vi "READ MODBUS DATA.vi"() -> ()   [LabVIEW 2025]
uses:
  <vilib>/NI/Modbus Library/API/Wrapper/Create TCP Master.vi
  <vilib>/NI/Modbus Library/API/Master/Modbus Master.lvclass
  <vilib>/NI/Modbus Library/API/Wrapper/API Main.lvlib
panel:
  out "Data Register":u16[](array[numeric])
  out "8":sgl
  out "7":sgl
  out "6":sgl
  out "5":sgl
  out "4":sgl
  out "3":sgl
  out "2":sgl
  out "1":sgl
  out "error out":errorcluster
  in  "Stop":bool
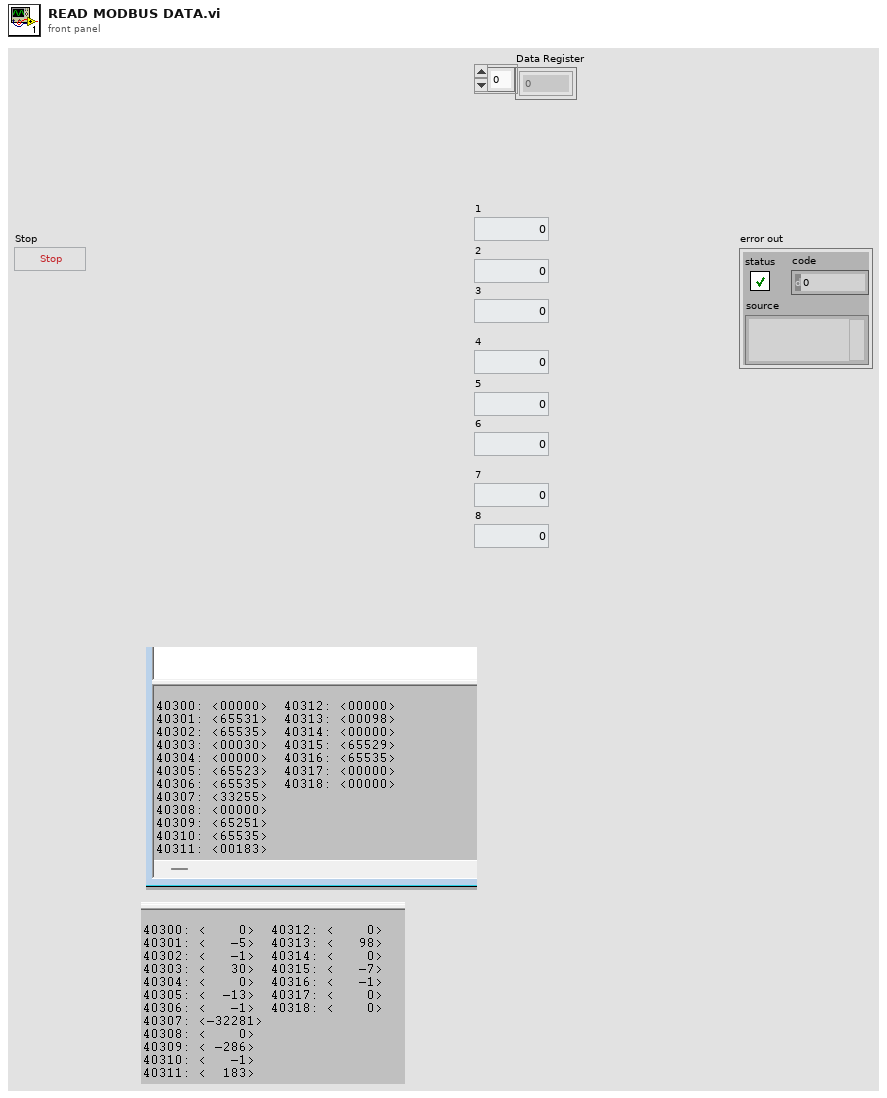
[diagram p1: front panel]
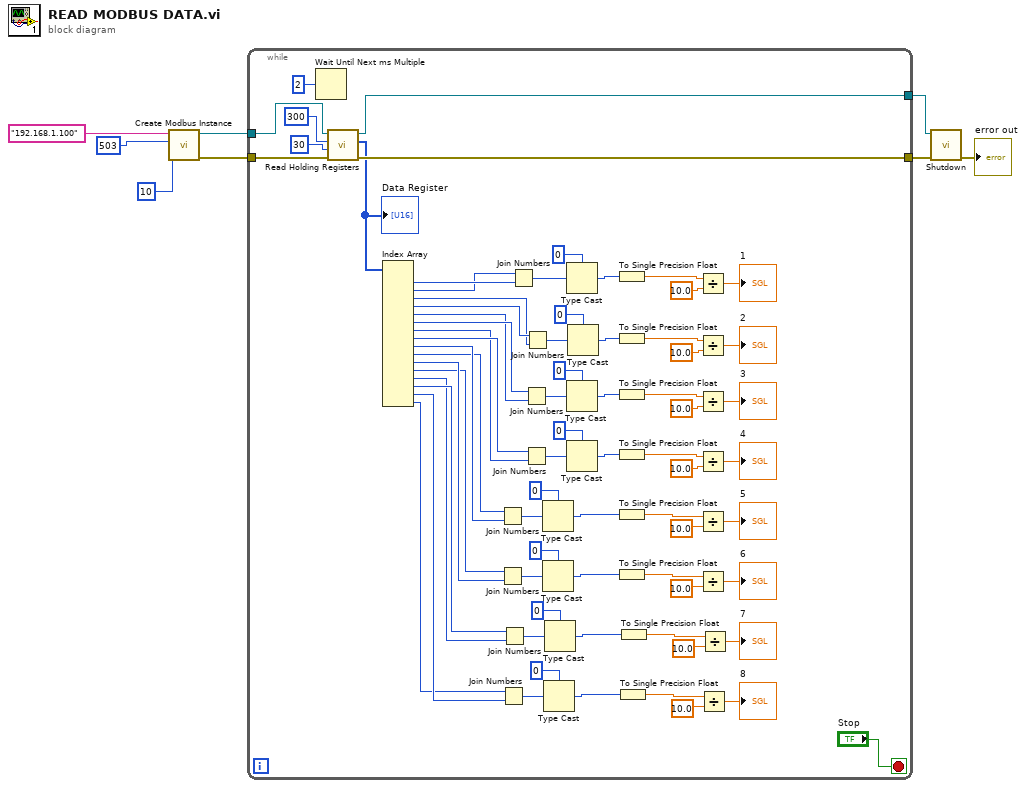
[diagram p0: block diagram]
diagram:
  n1 = call-poly <vilib>:"Create Modbus Instance.vi"("connect timeout ms"=10, "port (502)"=u16 503, "address"="192.168.1.100") -> ("error out"=w6:errorcluster, "TCP master instance"=w5:refnum<class "Modbus Master.lvclass">)  [unwired: 7 in]
  n2 = while {
    tunnel: w6 -> [w81]
    tunnel: w5 -> [w80]
    tunnel: [w75] -> w4
    tunnel: [w74] -> w3
    stop <- "Stop" stop-if-true
    n3 = Wait Until Next ms Multiple(millisecond multiple=u32 2) -> ()  [unwired: 1 out]
    n4 = call-dynamic "Read Holding Registers.vi"("error in"=w81, "number of inputs"=u16 30, "starting address"=u16 300, "Modbus master in"=w80) -> ("error out"=w75:errorcluster, "register values"=w65:u16[], "Modbus master out"=w74:refnum<class "Modbus Master.lvclass">)  [unwired: 5 in]
    "Data Register" <- w65
    n5 = Index Array(array=w65) -> (element #1=w67:u16, element #2=w66:u16, element #3=w57:u16, element #4=w58:u16, element #5=w49:u16, element #6=w50:u16, element #7=w41:u16, element #8=w42:u16, element #9=w34:u16, element #10=w33:u16, element #11=w26:u16, element #12=w25:u16, element #13=w17:u16, element #14=w18:u16, element #15=w10:u16, element #16=w9:u16)  [unwired: 16 in]
    n6 = Join Numbers(hi=w33, lo=w34) -> ((hi.lo)=w35:u32)
    n7 = Join Numbers(hi=w25, lo=w26) -> ((hi.lo)=w32:u32)
    n8 = Join Numbers(hi=w9, lo=w10) -> ((hi.lo)=w16:u32)
    n9 = Join Numbers(hi=w18, lo=w17) -> ((hi.lo)=w19:u32)
    n10 = Join Numbers(hi=w66, lo=w67) -> ((hi.lo)=w68:u32)
    n11 = Join Numbers(hi=w50, lo=w49) -> ((hi.lo)=w51:u32)
    n12 = Join Numbers(hi=w42, lo=w41) -> ((hi.lo)=w48:u32)
    n13 = Join Numbers(hi=w58, lo=w57) -> ((hi.lo)=w64:u32)
    n14 = Type Cast(type=0, x=w35) -> (*(type *) &x=w37:i32)
    n15 = Type Cast(type=0, x=w32) -> (*(type *) &x=w30:i32)
    n16 = Type Cast(type=0, x=w16) -> (*(type *) &x=w14:i32)
    n17 = Type Cast(type=0, x=w19) -> (*(type *) &x=w21:i32)
    n18 = Type Cast(type=0, x=w68) -> (*(type *) &x=w70:i32)
    n19 = Type Cast(type=0, x=w51) -> (*(type *) &x=w53:i32)
    n20 = Type Cast(type=0, x=w48) -> (*(type *) &x=w46:i32)
    n21 = Type Cast(type=0, x=w64) -> (*(type *) &x=w62:i32)
    n22 = To Single Precision Float(number=w70) -> (single precision float=w73:sgl)
    n23 = To Single Precision Float(number=w62) -> (single precision float=w59:sgl)
    n24 = To Single Precision Float(number=w53) -> (single precision float=w56:sgl)
    n25 = To Single Precision Float(number=w46) -> (single precision float=w43:sgl)
    n26 = To Single Precision Float(number=w37) -> (single precision float=w40:sgl)
    n27 = To Single Precision Float(number=w30) -> (single precision float=w27:sgl)
    n28 = To Single Precision Float(number=w14) -> (single precision float=w11:sgl)
    n29 = To Single Precision Float(number=w21) -> (single precision float=w24:sgl)
    n30 = Divide(x=w73, y=sgl 10.0) -> (x/y=→"1":sgl)
    n31 = Divide(x=w59, y=sgl 10.0) -> (x/y=→"2":sgl)
    n32 = Divide(x=w56, y=sgl 10.0) -> (x/y=→"3":sgl)
    n33 = Divide(x=w43, y=sgl 10.0) -> (x/y=→"4":sgl)
    n34 = Divide(x=w40, y=sgl 10.0) -> (x/y=→"5":sgl)
    n35 = Divide(x=w27, y=sgl 10.0) -> (x/y=→"6":sgl)
    n36 = Divide(x=w11, y=sgl 10.0) -> (x/y=→"8":sgl)
    n37 = Divide(x=w24, y=sgl 10.0) -> (x/y=→"7":sgl)
  }
  n38 = call-dynamic "Shutdown.vi"("error in"=w4, "Modbus master in"=w3) -> ("error out"=→"error out":errorcluster)  [unwired: 9 in]
